vi "Event handler-Z Setup.vi"(8 "error in (no error)":errorcluster, 9 "Obtain Z Stop":bool, 11 "Obtain Z Start":bool) -> (0 "error out":errorcluster)   [LabVIEW 2013]
uses:
  Typedefs/Read Write Enum.ctl
  Global Variables/gl_UI Ctrl Refs.vi
  Global Variables/General Globals.vi
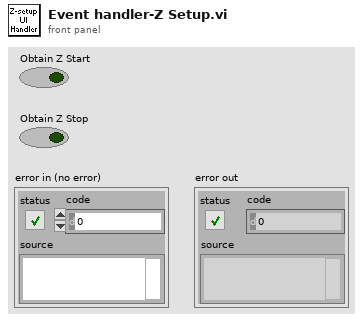
[diagram p1: front panel]
types:
  T1 = typedef "Read Write Enum.ctl" = enum16{"Read", "Write"}
  T2 = typedef "UI ctrl refs cluster.ctl" = cluster{"Top level VI path":path, "Top level VI ref":refnum<vi>, "User menu ref":refnum<k9>, "Sub Panel control":refnum<vi>, "Imaging Param Tab":refnum<vi>, "Occurrence-Start drivers":refnum<k4>, "Occurrence-Speed logging initialised":refnum<k4>, "Occurrence-XYZ stage initialised":refnum<k4>, "Exit button":refnum<vi>, "Status ind":refnum<vi>, "Return to Origin":refnum<vi>, "Speed Logging":refnum<vi>, "Time Lapse":refnum<vi>, "Live Imaging":refnum<vi>, "AOL Z Stack":refnum<vi>, "Motor Z Stack":refnum<vi>, "Funct Acq button":refnum<vi>, "Hard Shutter":refnum<vi>, "Virtual Shutter":refnum<vi>, "Laser Power":refnum<vi>, "AOL Mode":refnum<vi>, "Frame Size":refnum<vi>, "Field of View":refnum<vi>, "Dwell Time":refnum<vi>, "Zoom":refnum<vi>, "AOL Z":refnum<vi>, "Objective":refnum<vi>, "Axis":refnum<vi>, "Paths & Names":refnum<vi>, "Experiment folder path (ind.)":refnum<vi>, "Last State (Ind.)":refnum<vi>, "Laser wavelength ind (nm)":refnum<vi>, "Averages":refnum<vi>, "Angle (degrees)":refnum<vi>, "X centre":refnum<vi>, "Y centre":refnum<vi>, "Plane Mode":refnum<vi>, "# Planes":refnum<vi>, "Z Start":refnum<vi>, "Z Stop":refnum<vi>, "Z Step":refnum<vi>, "PMT 1":refnum<vi>, "PMT 2":refnum<vi>, "Stage XYZ Position":refnum<vi>, "Pockels@Z Start":refnum<vi>, "Pockels@Z Stop":refnum<vi>, "Obtain Z Start":refnum<vi>, "Obtain Z Stop":refnum<vi>, "Live stim.trig.period":refnum<vi>, "Live stim.trig.enable":refnum<vi>, "Funct. Acq. Pockels Modulation":refnum<vi>, "Enable Video Recording":refnum<vi>, "Video Record-Live Imaging":refnum<vi>, "Video Record-Funct acq":refnum<vi>, "AOL Z-stack Chirps Ready (ind)":refnum<vi>, "Center freq ind (nm)":refnum<vi>, "Logging queue (ind)":refnum<vi>, "Back aperture power (ind.)":refnum<vi>, "Power after objective (ind.)":refnum<vi>, "Switch user":refnum<vi>}
  T3 = typedef "Laser control knob.ctl" = u16
  T4 = cluster{"ZStack":cluster{"Zstart":dbl, "Zstop":dbl, "Zstep":dbl}, "Laser Power %":cluster{"@ Start":dbl, "@ Stop":dbl}}
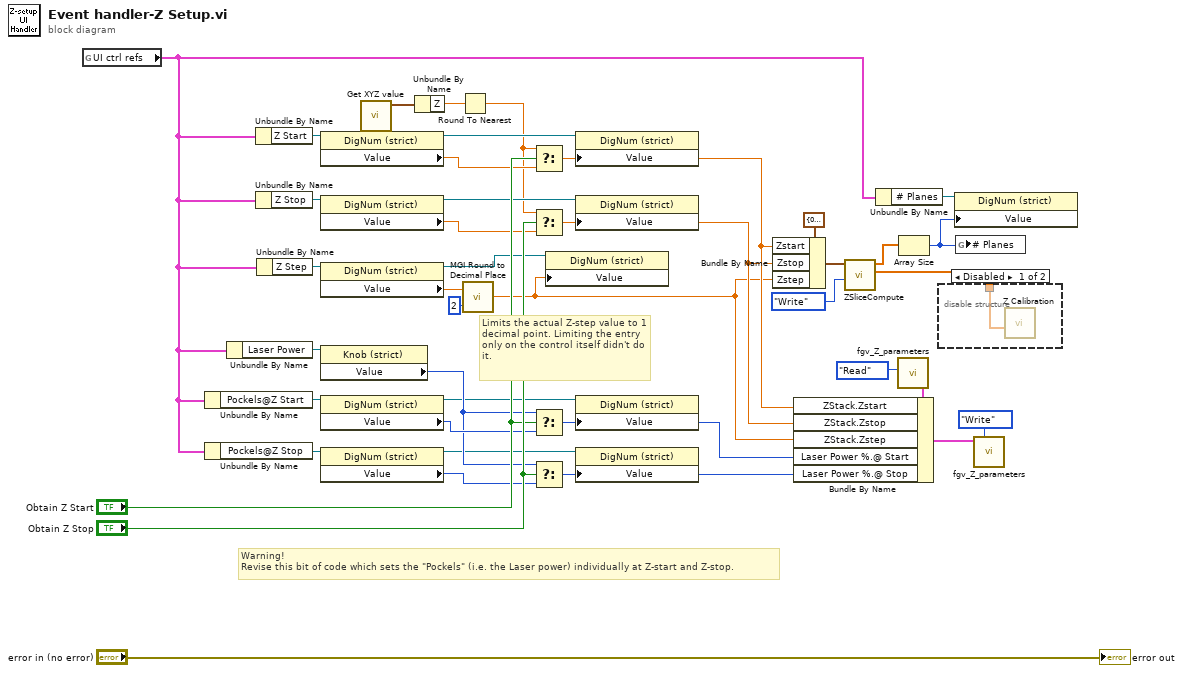
[diagram p0: block diagram]
diagram:
  # "Limits the actual Z-step value to 1 decimal point. Limiting the entry only on the control itself didn't do it."
  # "Warning!\nRevise this bit of code which sets the \"Pockels\" (i.e. the Laser power) individually at Z-start and Z-stop."
  n1 = global read "gl_UI Ctrl Refs.vi" "UI ctrl refs"() -> (w39:T2)
  n2 = Unbundle By Name(w39) -> ("Pockels@Z Start"=w16:refnum<vi>)
  n3 = Unbundle By Name(w39) -> ("Pockels@Z Stop"=w15:refnum<vi>)
  n4 = Unbundle By Name(w39) -> ("Laser Power"=w17:refnum<vi>)
  n5 = Unbundle By Name(w39) -> ("Z Start"=w23:refnum<vi>)
  n6 = Unbundle By Name(w39) -> ("Z Stop"=w22:refnum<vi>)
  n7 = Unbundle By Name(w39) -> ("Z Step"=w18:refnum<vi>)
  n8 = property on="Property Node" class="DigNum (strict)"(reference=w23) -> (reference out=w26:refnum<vi>, "Value"=w25:dbl)  [unwired: 1 in, 1 out]
  n9 = property on="Property Node" class="DigNum (strict)"(reference=w22) -> (reference out=w21:refnum<vi>, "Value"=w20:dbl)  [unwired: 1 in, 1 out]
  n10 = property on="Property Node" class="DigNum (strict)"(reference=w18) -> (reference out=w2:refnum<vi>, "Value"=w3:dbl)  [unwired: 1 in, 1 out]
  n11 = property on="Property Node" class="Knob (strict)"(reference=w17) -> ("Value"=w32:T3)  [unwired: 1 in, 2 out]
  n12 = property on="Property Node" class="DigNum (strict)"(reference=w16) -> (reference out=w14:refnum<vi>, "Value"=w33:u16)  [unwired: 1 in, 1 out]
  n13 = property on="Property Node" class="DigNum (strict)"(reference=w15) -> (reference out=w13:refnum<vi>, "Value"=w31:u16)  [unwired: 1 in, 1 out]
  n14 = call "Get XYZ value.vi"() -> ("Stage XYZ Position"=w7:cluster{"X":sgl, "Y":sgl, "Z":sgl})  [unwired: 11 in]
  n15 = Unbundle By Name(w7) -> ("Z"=w34:sgl)
  n16 = Round To Nearest(number=w34) -> (nearest integer value=w5:sgl)
  n17 = call "MGI Round to Decimal Place.vi"("Decimal Digits"=2, "Number"=w3) -> ("Rounded"=w1:dbl)  [unwired: 1 in]
  n18 = Select(t=w5, s="Obtain Z Start", f=w25) -> (s? t:f=w24:dbl)
  n19 = Select(t=w5, s="Obtain Z Stop", f=w20) -> (s? t:f=w19:dbl)
  n20 = Select(t=w32, s="Obtain Z Start", f=w33) -> (s? t:f=w12:T3)
  n21 = Select(t=w32, s="Obtain Z Stop", f=w31) -> (s? t:f=w11:T3)
  n22 = property on="Property Node" class="DigNum (strict)"(reference=w2, "Value"=w1) -> ()  [unwired: 1 in, 2 out]
  n23 = property on="Property Node" class="DigNum (strict)"(reference=w26, "Value"=w24) -> ()  [unwired: 1 in, 2 out]
  n24 = property on="Property Node" class="DigNum (strict)"(reference=w21, "Value"=w19) -> ()  [unwired: 1 in, 2 out]
  n25 = property on="Property Node" class="DigNum (strict)"(reference=w14, "Value"=w12) -> ()  [unwired: 1 in, 2 out]
  n26 = property on="Property Node" class="DigNum (strict)"(reference=w13, "Value"=w11) -> ()  [unwired: 1 in, 2 out]
  n27 = Bundle By Name(cluster=cluster{"Zstart":dbl, "Zstop":dbl, "Zstep":dbl} {"Zstart"=0.0, "Zstop"=0.0, "Zstep"=0.0} ("ZStack"), "Zstart"=w24, "Zstop"=w19, "Zstep"=w1) -> (w37:cluster{"Zstart":dbl, "Zstop":dbl, "Zstep":dbl})
  n28 = call "ZSliceCompute.vi"("Function"=Read_Write_Enum."Write", "ZStack (um)"=w37) -> ("AOL Z Planes(um)"=w35:dbl[], "Motor Z Planes(um)"=w36:dbl[])  [unwired: 6 in, 2 out]
  n29 = Unbundle By Name(w39) -> ("# Planes"=w10:refnum<vi>)
  n30 = call "fgv_Z_parameters.vi"("Function"=enum16{"Intialize", "Write", "Read", "Clear"}."Read") -> ("Z Parameters"=w28:T4)  [unwired: 9 in, 1 out]
  n31 = Bundle By Name(cluster=w28, "ZStack.Zstart"=w24, "ZStack.Zstop"=w19, "ZStack.Zstep"=w1, "Laser Power %.@ Start"=w12, "Laser Power %.@ Stop"=w11) -> (w27:T4)
  n32 = Array Size(array=w36) -> (size(s)=w8:i32)
  n33 = disable-structure "Diagram Disable Structure" shown="Disabled" {
    disable-tunnel: w35 -> [w42 _]
    frame Disabled {
      n34 = call "Z Calibration.vi"("Z Planes"=w42) -> ()  [unwired: 7 in, 4 out]
    }
    frame Enabled {
    }
  }
  n35 = property on="Property Node" class="DigNum (strict)"(reference=w10, "Value"=w8) -> ()  [unwired: 1 in, 2 out]
  n36 = global write "General Globals.vi" "# Planes"(w8) -> ()
  n37 = call "fgv_Z_parameters.vi"("Function"=enum16{"Intialize", "Write", "Read", "Clear"}."Write", "Z Parameters"=w27) -> ()  [unwired: 8 in, 2 out]
  "error out" <- "error in (no error)"
